vi "Change_Bits_in_Reg.vi"(0 "Reg Number":u16, 1 "Bit Number":u16, 2 "Word Length":u16, 3 "Bit Word In":u16, 4 "Reg In":u16[](array[numeric])) -> (5 "Reg Out":u16[](array[numeric]))   [LabVIEW 2011]
doc: "This VI lets you edit one or more bits in a single register selected from an array of registers. For example bits 4 to 6 in register 2 may set gain. This VI will allow you to easily edit only these bits.\n\nReg Number - this is the register number that will be edited. \n\nBit Number - this is the starting bit to be edited. If you want to edit bits 4 to 6, the bit number is 4.\n\nWord length - this is the number of bits that you want to edit. If you want to edit bits 4 to 6, the word length is 3.\n\nBit Word In - this is the new value for the bits being edited. If you want to change bit 4 to 6 to binary 101, you connect this input to 5."
panel:
  # "Input"
  # "Output"
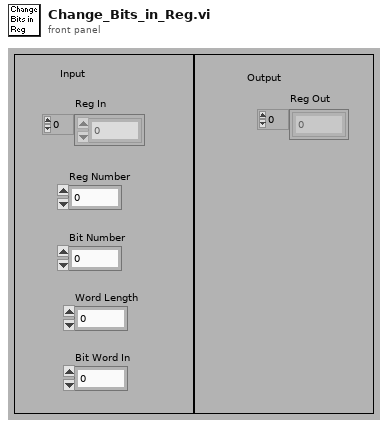
[diagram p1: front panel]
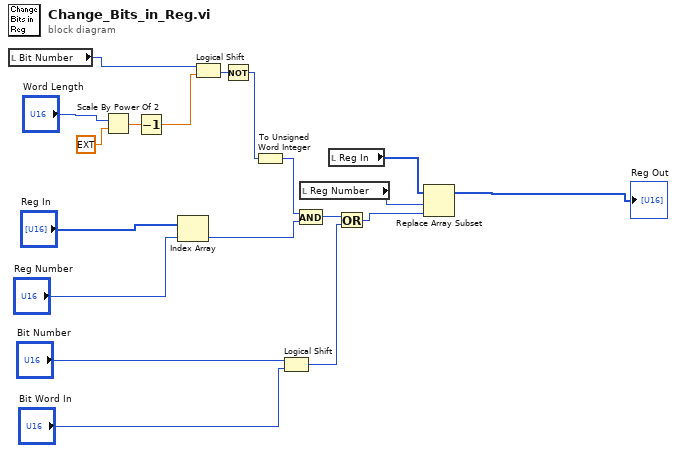
[diagram p0: block diagram]
diagram:
  n1 = local read "Bit Number"() -> (w3:u16)
  n2 = Scale By Power Of 2(n="Word Length", x=ext 1.0) -> (x*2^n=w17:ext)
  n3 = Decrement(x=w17) -> (x-1=w16:ext)
  n4 = Index Array(array="Reg In", index="Reg Number") -> (element=w12:u16)
  n5 = Logical Shift(y=w3, x=w16) -> (x << y=w1:u32)
  n6 = Not(x=w1) -> (.not. x?=w13:u32)
  n7 = To Unsigned Word Integer(number=w13) -> (unsigned 16bit integer=w14:u16)
  n8 = Logical Shift(y="Bit Number", x="Bit Word In") -> (x << y=w9:u16)
  n9 = And(x=w14, y=w12) -> (x .and. y?=w10:u16)
  n10 = local read "Reg Number"() -> (w18:u16)
  n11 = local read "Reg In"() -> (w19:u16[])
  n12 = Or(x=w10, y=w9) -> (x .or. y?=w11:u16)
  n13 = Replace Array Subset(array=w19, new element=w11, index=w18) -> (→"Reg Out":u16[])
